vi "Chose.vi"(8 "error in (no error)":errorcluster, 10 "Numeric":u32, 11 "CCD monitor in":refnum<class "CCD monitor.lvclass">) -> (0 "error out":errorcluster, 2 "element":refnum<class "CCD.lvclass">, 3 "CCD monitor out":refnum<class "CCD monitor.lvclass">)   [LabVIEW 2016, in "CCD monitor.lvlib" / "CCD monitor.lvclass"]
uses:
  <userlib>/Common Components/Hardware/Abstract System/Monitor/CCD monitor.lvclass
  <userlib>/Common Components/Hardware/CCD/CCD/CCD.lvclass
  <userlib>/Common Components/Hardware/Abstract System/Monitor/CCD monitor.lvclass/CCD monitor.ctl
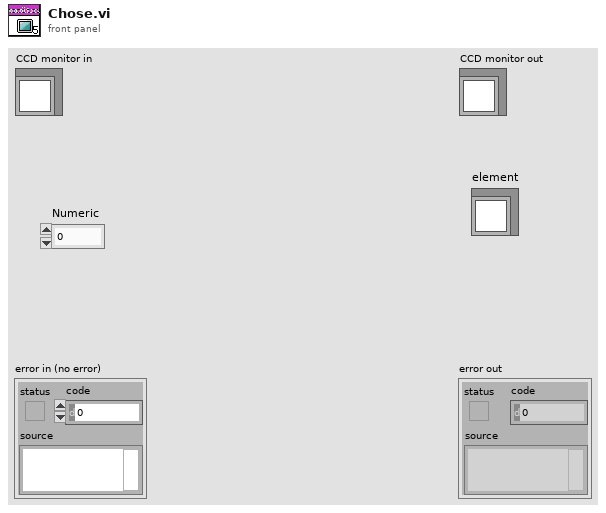
[diagram p1: front panel]
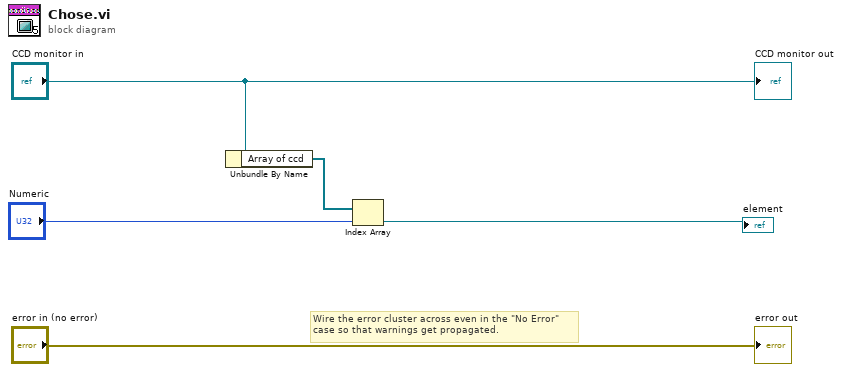
[diagram p0: block diagram]
diagram:
  # "Wire the error cluster across even in the \"No Error\"\ncase so that warnings get propagated."
  n1 = Unbundle By Name("CCD monitor in") -> ("Array of ccd"=w3:refnum<class "CCD.lvclass">[])
  n2 = Index Array(array=w3, index="Numeric") -> (element=→"element":refnum<class "CCD.lvclass">)
  "error out" <- "error in (no error)"
  "CCD monitor out" <- "CCD monitor in"
